vi "Obtain Session.vi"(8 "error in (no error)":errorcluster, 11 "Session  Name ()":string) -> (0 "error out":errorcluster, 3 "Session Handle":T1)   [LabVIEW 2018, in "Process Bar.lvclass"]
doc: "This function initializes the measurement\n\nPass the function a name to obtain an active measurement handle"
uses:
  Process Bar.lvclass
  Typedefs/Session Handle.ctl
  C:/Program Files/National Instruments/LabVIEW 2018/user.lib/_Session Fwk/Session - Root.lvclass
  Process Bar.lvclass/Process Bar.ctl
  <userlib>/_Session Fwk/Session - Root.lvclass
panel:
  in  "Status Msg":string
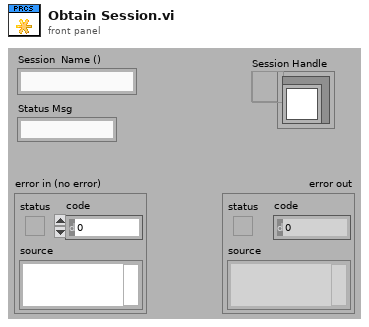
[diagram p1: front panel]
types:
  T1 = typedef "Process Bar.lvclass/Session Handle.ctl" = refnum<data-value>
  T2 = typedef "Session - Root.lvclass/Session Handle.ctl" = refnum<data-value>
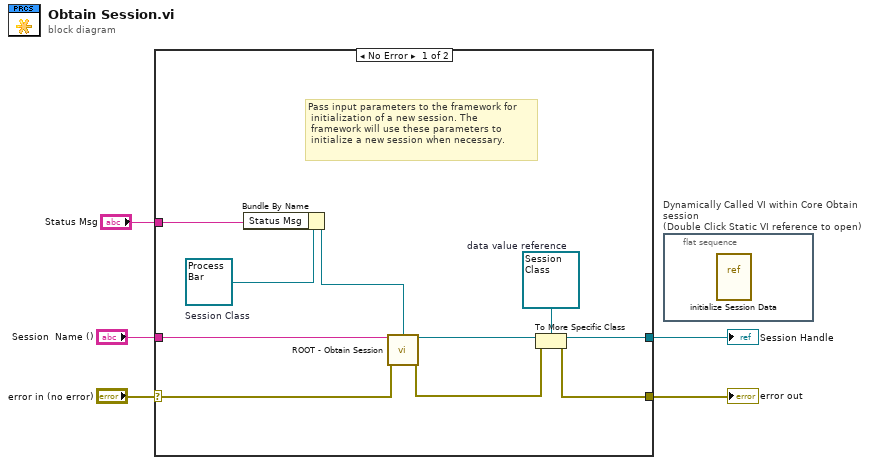
[diagram p0: block diagram]
diagram:
  n1 = case shown="No Error" "error in (no error)" {
    selector: "error in (no error)" -> [w14 w16]
    tunnel: [w11 w16] -> w4
    tunnel: [w13 _] -> w2
    tunnel: "Session  Name ()" -> [w15 _]
    tunnel: "Status Msg" -> [w6 _]
    frame No Error {
      w7 = refnum<data-value> refnum  # data value reference
      w8 = refnum<class "Process Bar.lvclass"> refnum  # Session Class
      # "Pass input parameters to the framework for\n initialization of a new session. The\n framework will use these parameters to\n initialize a new session when necessary."
      n2 = Bundle By Name(cluster=w8, "Status Msg"=w6) -> (w9:refnum<class "Process Bar.lvclass">)
      n3 = call <userlib>:"ROOT - Obtain Session.vi"("Session Name ()"=w15, "OBJ - Session"=w9, "error in (no error)"=w14) -> ("Session Handle"=w10:T2, "error out"=w12:errorcluster)  [unwired: 10 in, 1 out]
      n4 = To More Specific Class(target class=w7, reference=w10, error in=w12) -> (specific class reference=w13:refnum<data-value>, error out=w11:errorcluster)
    }
    frame Error {
    }
  }
  "error out" <- w4
  "Session Handle" <- w2
  n5 = flat-sequence "Dynamically Called VI within Core Obtain session\n(Double Click Static VI reference to open)" {
    frame #0 {
      n6 = vi-ref "initialize Session Data.vi"() -> ()  [unwired: 1 out]
    }
  }
